vi "terminal voltage readbacks.vi"() -> ()   [LabVIEW 2016, in "features.lvlib"]
doc: "This vi uses the control room rio to readback the terminal voltage settings. It must have the control room rio in the project to run correctly"
uses:
  Features/features/features.lvlib
panel:
  out "sum":dbl format="%#.3g"
  out "Grid":dbl format="%#.3g"
  out "error out":errorcluster
  in  "stop":bool
  out "Le Chain":dbl format="%#.3g"
  out "Le Column":dbl format="%#.3g"
  out "Le IND":dbl format="%.2f"
  out "LE Supp":dbl format="%.2f"
  out "He Chain":dbl format="%#.3g"
  out "HE Column":dbl format="%#.2g"
  out "He ind":dbl format="%.2f"
  out "He Supp":dbl format="%#.5g"
  out "Corona Current":dbl format="%#.3g"
  out "Terminal voltage":dbl format="%#.3g"
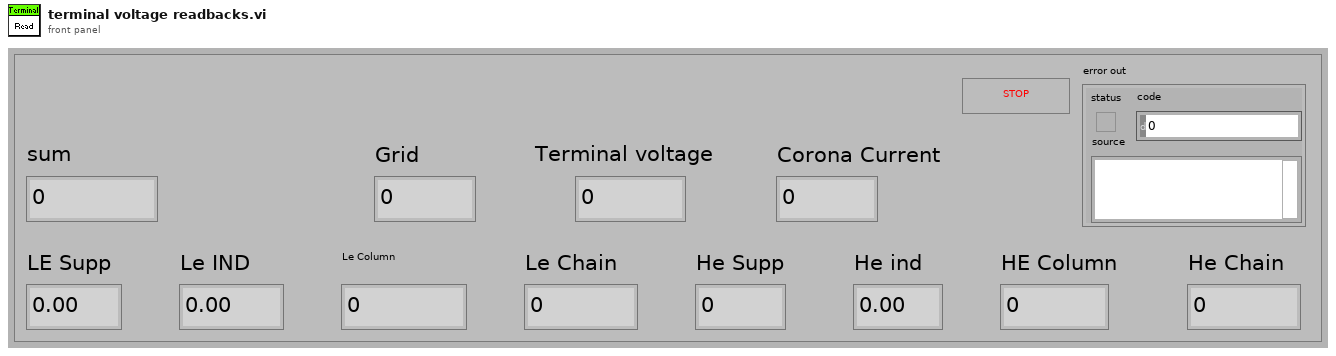
[diagram p1: front panel]
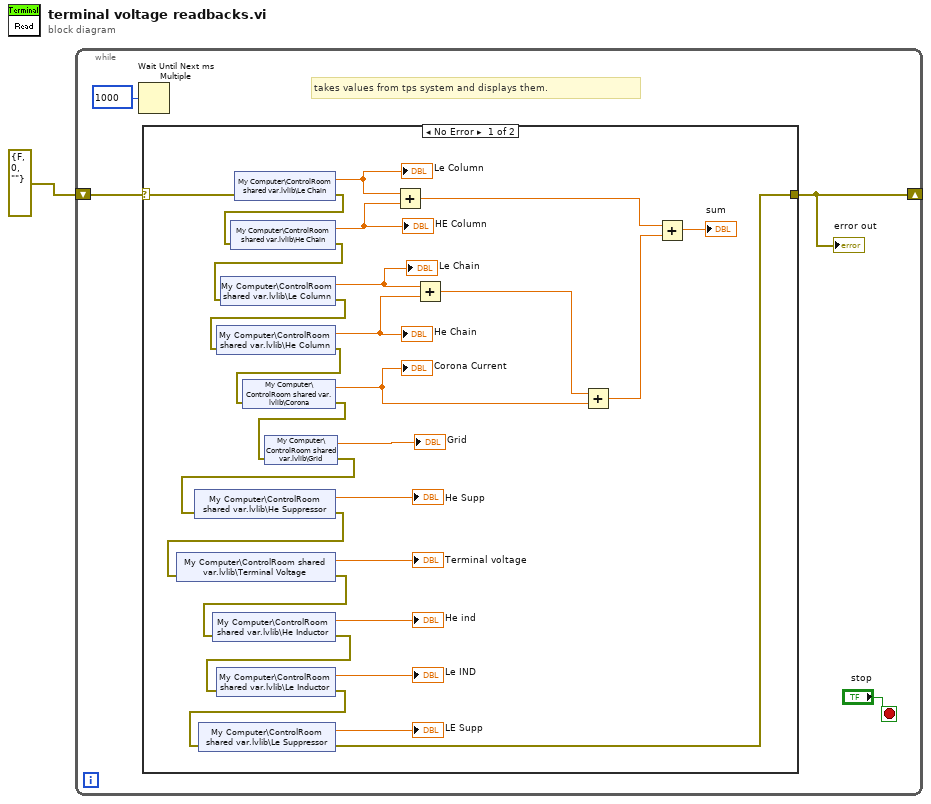
[diagram p0: block diagram]
diagram:
  n1 = while {
    shift-right: [w2] -> _
    shift-left: errorcluster {"status"=FALSE, "code"=0, "source"=""} ("error in (no error)") -> [w3]
    stop <- "stop" stop-if-true
    # "takes values from tps system and displays them."
    n2 = Wait Until Next ms Multiple(millisecond multiple=u32 1000) -> ()  [unwired: 1 out]
    n3 = case shown="No Error" w3 {
      selector: w3 -> [w6 w33]
      tunnel: [w32 w33] -> w2
      frame No Error {
        n4 = shared-variable "My Computer\\ControlRoom shared var.lvlib\\Le Chain"(error in=w6) -> (w28:dbl, error out=w7:errorcluster)
        "Le Column" <- w28
        n5 = shared-variable "My Computer\\ControlRoom shared var.lvlib\\He Chain"(error in=w7) -> (w14:dbl, error out=w8:errorcluster)
        "HE Column" <- w14
        n6 = shared-variable "My Computer\\ControlRoom shared var.lvlib\\Le Column"(error in=w8) -> (w13:dbl, error out=w9:errorcluster)
        "Le Chain" <- w13
        n7 = shared-variable "My Computer\\ControlRoom shared var.lvlib\\He Column"(error in=w9) -> (w23:dbl, error out=w10:errorcluster)
        "He Chain" <- w23
        n8 = shared-variable "My Computer\\ControlRoom shared var.lvlib\\Corona"(error in=w10) -> (w22:dbl, error out=w11:errorcluster)
        "Corona Current" <- w22
        n9 = shared-variable "My Computer\\ControlRoom shared var.lvlib\\Grid"(error in=w11) -> (→"Grid":dbl, error out=w12:errorcluster)
        n10 = shared-variable "My Computer\\ControlRoom shared var.lvlib\\He Suppressor"(error in=w12) -> (→"He Supp":dbl, error out=w17:errorcluster)
        n11 = shared-variable "My Computer\\ControlRoom shared var.lvlib\\Terminal Voltage"(error in=w17) -> (→"Terminal voltage":dbl, error out=w20:errorcluster)
        n12 = shared-variable "My Computer\\ControlRoom shared var.lvlib\\He Inductor"(error in=w20) -> (→"He ind":dbl, error out=w19:errorcluster)
        n13 = shared-variable "My Computer\\ControlRoom shared var.lvlib\\Le Inductor"(error in=w19) -> (→"Le IND":dbl, error out=w18:errorcluster)
        n14 = shared-variable "My Computer\\ControlRoom shared var.lvlib\\Le Suppressor"(error in=w18) -> (→"LE Supp":dbl, error out=w32:errorcluster)
        n15 = Add(x=w28, y=w14) -> (x+y=w15:dbl)
        n16 = Add(x=w13, y=w23) -> (x+y=w21:dbl)
        n17 = Add(x=w21, y=w22) -> (x+y=w16:dbl)
        n18 = Add(x=w15, y=w16) -> (x+y=→"sum":dbl)
      }
      frame Error {
      }
    }
    "error out" <- w2
  }
